vi "Keyence.Main.Close.vi"(8 "error in":errorcluster, 11 "Data in":T1={"Status"={"State"=enum."Init", "Ref"=refnum, "Bank"=0, "Version"="", "Model"="", "EndTS"=timestamp(0 s since 1904-01-01), "ImgPath"=path ""}, "Sets"={"IP"="192.168.2.1", "Timeout_ms"=5000, "Retries"=0, "ReconnectPeriod_s"=0, "ResetPeriod_s"=0, "ReadImg"=FALSE}, "Code"={"text"="", "status"=FALSE, "corners"=[], "level"=0, "class"="", "path"=path ""}}) -> (0 "error out":errorcluster, 3 "Data out":T1={"Status"={"State"=enum."Init", "Ref"=refnum, "Bank"=0, "Version"="", "Model"="", "EndTS"=timestamp(0 s since 1904-01-01), "ImgPath"=path ""}, "Sets"={"IP"="192.168.2.1", "Timeout_ms"=5000, "Retries"=0, "ReconnectPeriod_s"=0, "ResetPeriod_s"=0, "ReadImg"=FALSE}, "Code"={"text"="", "status"=FALSE, "corners"=[], "level"=0, "class"="", "path"=path ""}})   [LabVIEW 2015]
uses:
  Keyence.Data.ctl
  Keyence.Data.Status.ctl
  Keyence.Data.Status.State.ctl
  Keyence.Data.Sets.ctl
  LowLevel/Keyence.CodeDetails.ctl
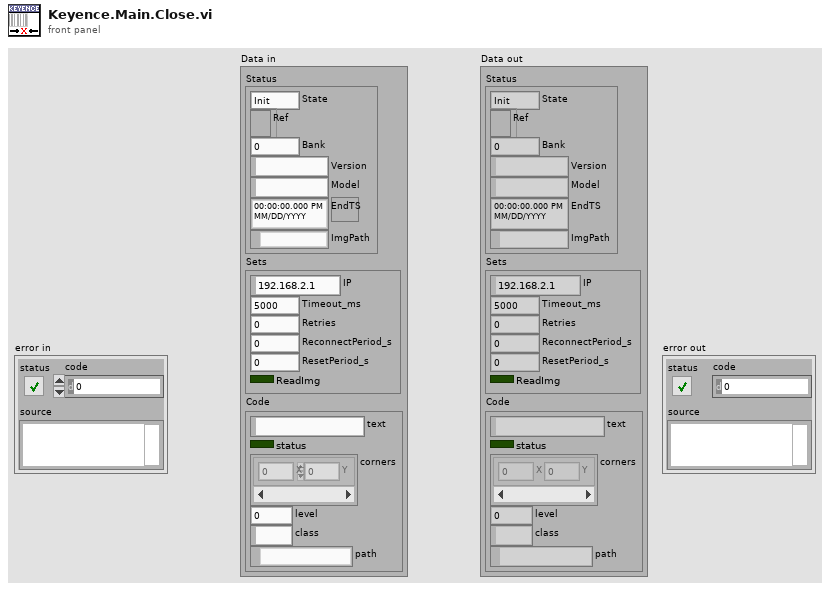
[diagram p1: front panel]
types:
  T1 = typedef "Keyence.Data.ctl" = cluster{"Status":T2, "Sets":T4, "Code":T5}
  T2 = typedef "Keyence.Data.Status.ctl" = cluster{"State":T3, "Ref":refnum<k5>, "Bank":u8, "Version":string, "Model":string, "EndTS":timestamp, "ImgPath":path}
  T3 = typedef "Keyence.Data.Status.State.ctl" = enum16{"First", "Init", "Reset", "Idle", "Scan"}
  T4 = typedef "Keyence.Data.Sets.ctl" = cluster{"IP":string, "Timeout_ms":i32, "Retries":i32, "ReconnectPeriod_s":i32, "ResetPeriod_s":i32, "ReadImg":bool}
  T5 = typedef "Keyence.CodeDetails.ctl" = cluster{"text":string, "status":bool, "corners":cluster{"X":i32, "Y":i32}[], "level":u8, "class":string, "path":path}
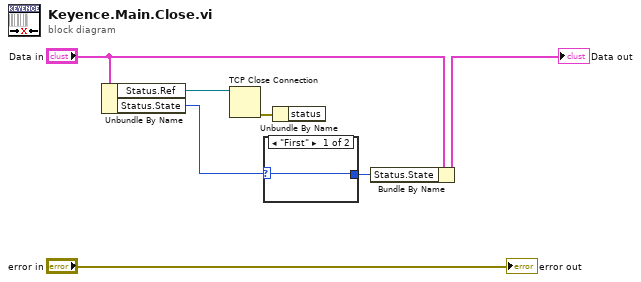
[diagram p0: block diagram]
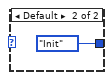
[diagram p2: hidden frame]
diagram:
  n1 = Unbundle By Name("Data in") -> ("Status.Ref"=w2:refnum<k5>, "Status.State"=w1:T3)
  n2 = TCP Close Connection(connection ID=w2) -> (error out=w3:errorcluster)  [unwired: 2 in, 1 out]
  n3 = case shown="\"First\"" w1 {
    selector: w1 -> [w8 _]
    tunnel: [w8 Keyence.Data.Status.State."Init" ("State (Init)")] -> w6
    frame "First" {
    }
    frame Default {
    }
  }
  n4 = Unbundle By Name(w3) -> ()  [unwired: 1 out]
  n5 = Bundle By Name(cluster="Data in", "Status.State"=w6) -> (→"Data out":T1)
  "error out" <- "error in"
